vi "Resize Panel to Pane.vi"(8 "error in (no error)":errorcluster, 10 "Apply Recursively? (F)":bool, 11 "MediatorBusMonitor In":refnum<class "MediatorBusMonitor.lvclass">) -> (0 "error out":errorcluster, 3 "MediatorBusMonitor Out":refnum<class "MediatorBusMonitor.lvclass">)   [LabVIEW 2017, in "Mediator.lvlib" / "MediatorBusMonitor.lvclass"]
doc: "<License>\nCopyright © 2017 Composed Systems, LLC | All rights reserved\nwww.composed.io\n\nAuthor: Ethan Stern <ethan.stern@composed.io>\n\nThis software is provided \"AS IS\" WITHOUT WARRANTIES, either express or implied, AND IS FOR EDUCATIONAL PURPOSES ONLY.\n</License>"
uses:
  MediatorBusMonitor.lvclass
  MediatorBusMonitor.lvclass/MediatorBusMonitor.ctl
  gpm_packages/@cs/listbox/Source/ListboxExtensions.lvlib
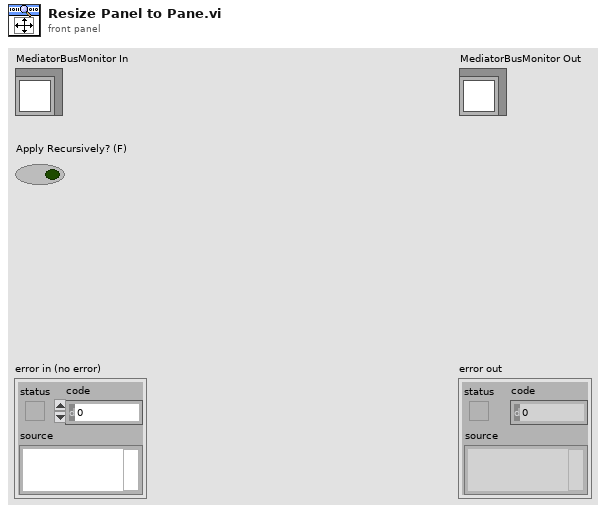
[diagram p1: front panel]
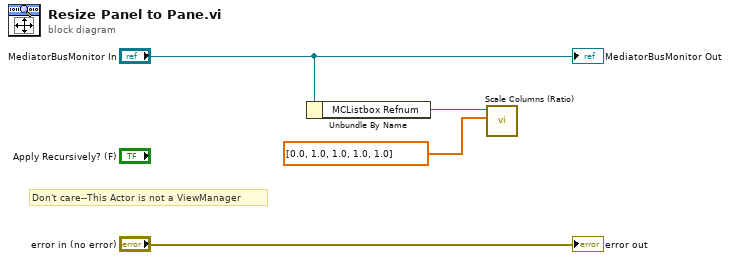
[diagram p0: block diagram]
diagram:
  # "Don't care--This Actor is not a ViewManager"
  n1 = Unbundle By Name("MediatorBusMonitor In") -> ("MCListbox Refnum"=w2:refnum<vi>)
  n2 = call "Scale Columns (Ratio).vi"("Column Widths [unitless ratio]"=dbl[] [0.0, 1.0, 1.0, 1.0, 1.0], "MulticolumnListbox in"=w2) -> ()  [unwired: 9 in, 1 out]
  "error out" <- "error in (no error)"
  "MediatorBusMonitor Out" <- "MediatorBusMonitor In"
